vi "数值显示转换.vi"(7 "显示":refnum<vi>, 11 "数组":T1(array[cluster])) -> ()   [LabVIEW 2016]
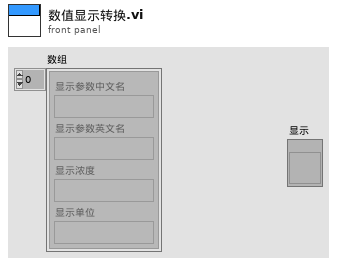
[diagram p1: front panel]
types:
  T1 = cluster{"显示参数中文名":string, "显示参数英文名":string, "显示浓度":string, "显示单位":string}[]
  T2 = cluster{"显示参数中文名":string, "显示参数英文名":string, "显示浓度":string, "显示单位":string}
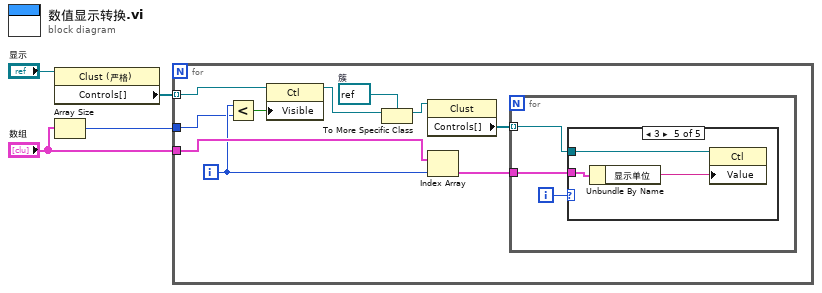
[diagram p0: block diagram]
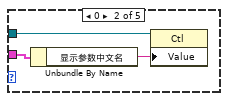
[diagram p3: hidden frame]
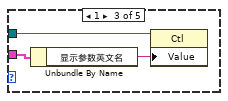
[diagram p4: hidden frame]
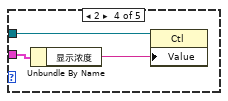
[diagram p5: hidden frame]
diagram:
  n1 = property class="Clust (严格)"(reference="显示") -> ("Controls[]"=w3:refnum<vi>[])  [unwired: 1 in, 2 out]
  n2 = Array Size(array="数组") -> (size(s)=w1:i32)
  n3 = for {
    tunnel: w3 -> [w13] mode=indexing
    tunnel: "数组" -> [w14]
    tunnel: w1 -> [w7]
    i -> [w8]
    w12 = refnum<vi> refnum  # 簇
    n4 = Less?(x=w8, y=w7) -> (x < y?=w5:bool)
    n5 = property class="Ctl"(reference=w13, "Visible"=w5) -> (reference out=w6:refnum<vi>)  [unwired: 1 in, 1 out]
    n6 = To More Specific Class(target class=w12, reference=w6) -> (specific class reference=w11:refnum<vi>)  [unwired: 1 in, 1 out]
    n7 = property class="Clust"(reference=w11) -> ("Controls[]"=w10:refnum<vi>[])  [unwired: 1 in, 2 out]
    n8 = Index Array(array=w14, index=w8) -> (element=w9:T2)
    n9 = for {
      tunnel: w10 -> [w16] mode=indexing
      tunnel: w9 -> [w15]
      i -> [w17]
      n10 = case shown="3" w17 {
        tunnel: w16 -> [_ w20 w23 w26 w29]
        tunnel: w15 -> [_ w19 w22 w25 w28]
        frame Default {
        }
        frame 0 {
          n11 = Unbundle By Name(w19) -> ("显示参数中文名"=w18:string)
          n12 = property class="Ctl"(reference=w20, "Value"=w18) -> ()  [unwired: 1 in, 2 out]
        }
        frame 1 {
          n13 = Unbundle By Name(w22) -> ("显示参数英文名"=w21:string)
          n14 = property class="Ctl"(reference=w23, "Value"=w21) -> ()  [unwired: 1 in, 2 out]
        }
        frame 2 {
          n15 = Unbundle By Name(w25) -> ("显示浓度"=w24:string)
          n16 = property class="Ctl"(reference=w26, "Value"=w24) -> ()  [unwired: 1 in, 2 out]
        }
        frame 3 {
          n17 = Unbundle By Name(w28) -> ("显示单位"=w27:string)
          n18 = property class="Ctl"(reference=w29, "Value"=w27) -> ()  [unwired: 1 in, 2 out]
        }
      }
    }
  }
